vi "Confirm Action.vi"(8 "Confirm":bool, 9 "Dump All":bool) -> (4 "The Indicator":bool)   [LabVIEW 2014]
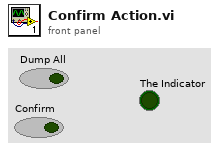
[diagram p1: front panel]
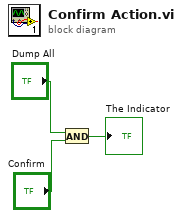
[diagram p0: block diagram]
diagram:
  n1 = And(x="Dump All", y="Confirm") -> (x .and. y?=→"The Indicator":bool)
